vi "find labview exe.vi"(8 "error in":errorcluster, 11 "desired lv version":dbl) -> (0 "error out":errorcluster, 3 "labview directory":path)   [LabVIEW 2013]
uses:
  <vilib>/Utility/sysdir.llb/Get System Directory.vi
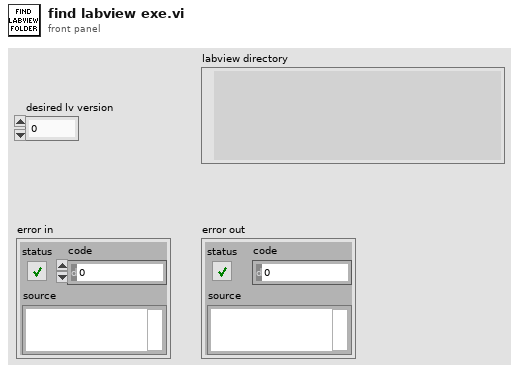
[diagram p1: front panel]
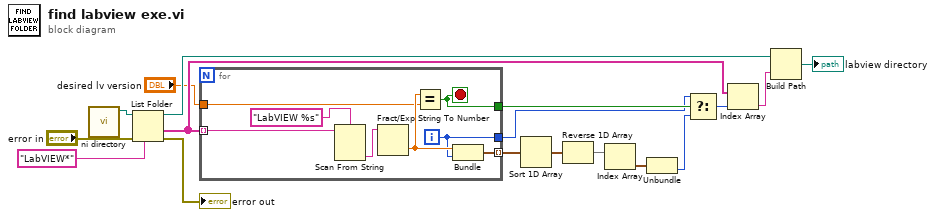
[diagram p0: block diagram]
diagram:
  n1 = call "ni directory.vi"() -> ("National Instruments"=w6:path)  [unwired: 11 in]
  n2 = List Folder(path=w6, pattern="LabVIEW*", error in="error in") -> (path out=w13:path, folder names=w15:string[], error out=→"error out":errorcluster)  [unwired: 1 in, 1 out]
  n3 = for {
    tunnel: w15 -> [w25] mode=indexing
    tunnel: [w20] -> w8 mode=indexing
    tunnel: "desired lv version" -> [w21]
    tunnel: [w19] -> w2
    tunnel: [w18] -> w1
    i -> [w18]
    stop <- w19 stop-if-true
    n4 = Scan From String(format string="LabVIEW %s", input string=w25) -> (output 1=w23:string)  [unwired: 3 in, 3 out]
    n5 = Fract/Exp String To Number(string=w23) -> (number=w22:dbl)  [unwired: 3 in, 1 out]
    n6 = Equal?(x=w22, y=w21) -> (x = y?=w19:bool)
    n7 = Bundle(w22, w18) -> (w20:cluster{dbl, i32})  [unwired: 1 in]
  }
  n8 = Sort 1D Array(array=w8) -> (sorted array=w9:cluster{dbl, i32}[])
  n9 = Reverse 1D Array(array=w9) -> (reversed array=w12:cluster{dbl, i32}[])
  n10 = Index Array(array=w12) -> (element=w10:cluster{dbl, i32})  [unwired: 1 in]
  n11 = Unbundle(w10) -> (w11:i32)  [unwired: 1 out]
  n12 = Select(t=w1, s=w2, f=w11) -> (s? t:f=w3:i32)
  n13 = Index Array(array=w15, index=w3) -> (element=w14:string)
  n14 = Build Path(base path=w13, name or relative path=w14) -> (appended path=→"labview directory":path)
